vi "ReadRelHumidity.vi"(6 "Error In":errorcluster, 8 "Cluster":T1, 9 "LINX Resource":T2={"IO"=enum."Remote", "Interface"=enum."Serial", "LINX Device Config"={"Interface"=enum."Serial", "COM Port"="COM13", "TCP Configuration"={"IP Address"="", "Port"=0}, "Device Family"=1, "Device ID"=1, "Device Name"="myRIO-1900", "TCP Ref"=refnum, "Channels"={"DI"=[0, 1, 2, 3, 4, 5, 6, 7, 8, 9, 10, 11, 12, 13, 14, 15, 16, 17, 18, 19, 20, 21, 22, 23, 24, 25, 26, 27, 28, 29, 30, 31, 32, 33, 34, 35, 36, 37, 38, 39, 40, 41, 42, 43, 44, 45, 46], "DO"=[0, 1, 2, 3, 4, 5, 6, 7, 8, 9, 10, 11, 12, 13, 14, 15, 16, 17, 18, 19, 20, 21, 22, 23, 24, 25, 26, 27, 28, 29, 30, 31, 32, 33, 34, 35, 36, 37, 38, 39, 40, 41, 42, 43, 44, 45, 46], "AI"=[0, 1, 2, 3, 4, 5, 6, 7, 8, 9, 10, 11], "AO"=[], "PWM"=[3, 5, 6, 9, 10], "QE"=[], "UART"=[0, 1], "I2C 2"=[0], "SPI"=[0], "CAN"=[], "Servo"=[], "AI Ref (V)"=0.0, "AI Resolution (Bits)"=0, "AO Ref (V)"=0.0, "AO Resolution (Bits)"=0}}}) -> (0 "Error Out":errorcluster, 1 "Data RH":dbl[](array[numeric]), 2 "RH":dbl, 3 "LINX Resource":T2={"IO"=enum."Remote", "Interface"=enum."Serial", "LINX Device Config"={"Interface"=enum."Serial", "COM Port"="COM13", "TCP Configuration"={"IP Address"="", "Port"=0}, "Device Family"=1, "Device ID"=1, "Device Name"="myRIO-1900", "TCP Ref"=refnum, "Channels"={"DI"=[0, 1, 2, 3, 4, 5, 6, 7, 8, 9, 10, 11, 12, 13, 14, 15, 16, 17, 18, 19, 20, 21, 22, 23, 24, 25, 26, 27, 28, 29, 30, 31, 32, 33, 34, 35, 36, 37, 38, 39, 40, 41, 42, 43, 44, 45, 46], "DO"=[0, 1, 2, 3, 4, 5, 6, 7, 8, 9, 10, 11, 12, 13, 14, 15, 16, 17, 18, 19, 20, 21, 22, 23, 24, 25, 26, 27, 28, 29, 30, 31, 32, 33, 34, 35, 36, 37, 38, 39, 40, 41, 42, 43, 44, 45, 46], "AI"=[0, 1, 2, 3, 4, 5, 6, 7, 8, 9, 10, 11], "AO"=[], "PWM"=[3, 5, 6, 9, 10], "QE"=[], "UART"=[0, 1], "I2C 2"=[0], "SPI"=[0], "CAN"=[], "Servo"=[], "AI Ref (V)"=0.0, "AI Resolution (Bits)"=0, "AO Ref (V)"=0.0, "AO Resolution (Bits)"=0}}})   [LabVIEW 2024]
uses:
  <vilib>/MakerHub/LINX/Private/Type Defs/LINX Ref.ctl
  <vilib>/MakerHub/LINX/Private/Type Defs/Platform.ctl
  <vilib>/MakerHub/LINX/Private/Type Defs/Interface.ctl
  <vilib>/MakerHub/LINX/Private/Device/Type Defs/LINX Device Config.ctl
  <vilib>/MakerHub/LINX/Private/Device/Type Defs/TCP Config.ctl
  <vilib>/MakerHub/LINX/Private/Device/Type Defs/Channels.ctl
  <vilib>/MakerHub/LINX/Private/Local IO/LinxI2cWrite.vi
  <vilib>/MakerHub/LINX/Public/Utilities/Check Channel.vi
  <vilib>/MakerHub/LINX/Private/Local IO/Handle Errors.vi
  <vilib>/MakerHub/LINX/Private/Utilties/Generate Error.vi
  <vilib>/MakerHub/LINX/LMH-LINX.lvlib
  <vilib>/MakerHub/LINX/Private/Device/Device.lvlib
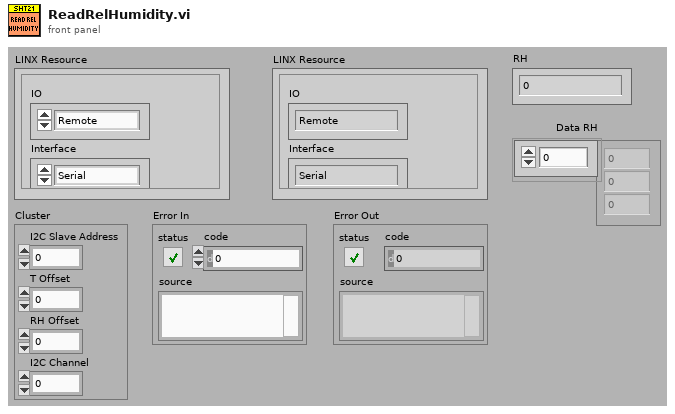
[diagram p1: front panel]
types:
  T1 = cluster{"I2C Slave Address":u8, "T Offset":dbl, "RH Offset":dbl, "I2C Channel":u8}
  T2 = typedef "LMH-LINX.lvlib/LINX Ref.ctl" = cluster{"IO":T3, "Interface":T4, "LINX Device Config":T5}
  T3 = typedef "LMH-LINX.lvlib/Platform.ctl" = enum16{"Remote", "Local"}
  T4 = typedef "LMH-LINX.lvlib/Interface.ctl" = enum16{"Serial", "TCP"}
  T5 = typedef "LMH-LINX.lvlib/Device.lvlib/LINX Device Config.ctl" = cluster{"Interface":T4, "COM Port":refnum<visa-resource-name>, "TCP Configuration":T6, "Device Family":u8, "Device ID":u8, "Device Name":string, "TCP Ref":refnum<k5>, "Channels":T7}
  T6 = typedef "LMH-LINX.lvlib/Device.lvlib/TCP Config.ctl" = cluster{"IP Address":string, "Port":u16}
  T7 = typedef "LMH-LINX.lvlib/Channels.ctl" = cluster{"DI":u8[], "DO":u8[], "AI":u8[], "AO":u8[], "PWM":u8[], "QE":u8[], "UART":u8[], "I2C 2":u8[], "SPI":u8[], "CAN":u8[], "Servo":u8[], "AI Ref (V)":dbl, "AI Resolution (Bits)":u8, "AO Ref (V)":dbl, "AO Resolution (Bits)":u8}
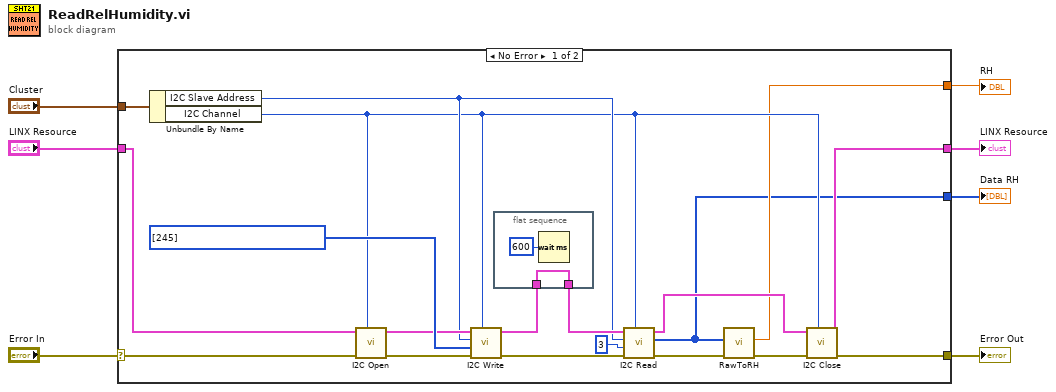
[diagram p0: block diagram]
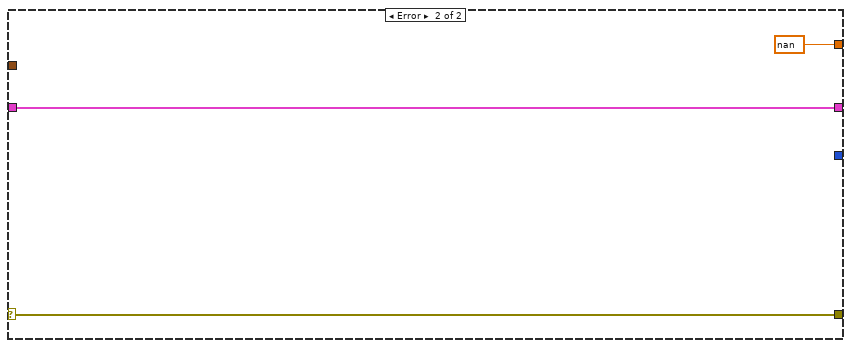
[diagram p2: hidden frame]
diagram:
  n1 = case shown="No Error" "Error In" {
    selector: "Error In" -> [w11 w31]
    tunnel: [w25 w31] -> w3
    tunnel: "LINX Resource" -> [w26 w30]
    tunnel: [w24 w30] -> w6
    tunnel: [w12 nan] -> w5
    tunnel: [w8 _] -> w4
    tunnel: "Cluster" -> [w10 _]
    frame No Error {
      n2 = Unbundle By Name(w10) -> ("I2C Slave Address"=w14:u8, "I2C Channel"=w13:u8)
      n3 = call <vilib>:"I2C Open.vi"("I2C Channel (0)"=w13, "Error In"=w11, "LINX Resource"=w26) -> ("Error Out"=w15:errorcluster, "LINX Resource"=w22:T2)  [unwired: 7 in]
      n4 = call <vilib>:"I2C Write.vi"("I2C Channel"=w13, "Error In"=w15, "Data"=u8[] [245], "I2C Slave Address (0)"=w14, "LINX Resource"=w22) -> ("Error Out"=w20:errorcluster, "LINX Resource"=w17:T2)  [unwired: 5 in]
      n5 = flat-sequence {
        tunnel: [w28] -> w16
        tunnel: w17 -> [w28]
        frame #0 {
          n6 = Wait (ms)(milliseconds to wait=u32 600) -> ()  [unwired: 1 out]
        }
      }
      n7 = call <vilib>:"I2C Read.vi"("I2C Channel"=w13, "Error In"=w20, "Bytes To Read"=u8 3, "I2C Slave Address (0)"=w14, "LINX Resource"=w16) -> ("Error Out"=w9:errorcluster, "Data"=w8:u8[], "LINX Resource"=w18:T2)  [unwired: 4 in]
      n8 = call "RawToRH.vi"("Error In"=w9, "Data"=w8) -> ("Error Out"=w19:errorcluster, "RH"=w12:dbl)  [unwired: 6 in]
      n9 = call <vilib>:"I2C Close.vi"("I2C Channel (0)"=w13, "Error In"=w19, "LINX Resource"=w18) -> ("Error Out"=w25:errorcluster, "LINX Resource"=w24:T2)  [unwired: 7 in]
    }
    frame Error {
    }
  }
  "LINX Resource" <- w6
  "RH" <- w5
  "Data RH" <- w4
  "Error Out" <- w3
